vi "CopyOneBlock.vi"(8 "error in (no error)":errorcluster, 10 "block":u16) -> (0 "error out":errorcluster, 1 "data 2":u16[](array[numeric]), 2 "data 1":u16[](array[numeric]))   [LabVIEW 2015, in "ESLSCDLL.lvlib"]
uses:
  ESLSCDLL.lvlib
  Globals.vi
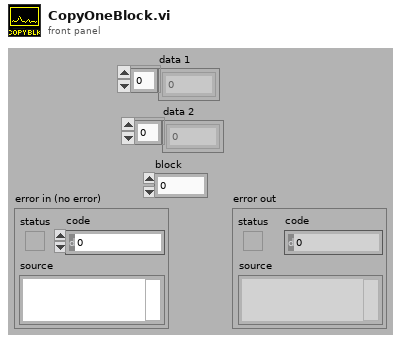
[diagram p1: front panel]
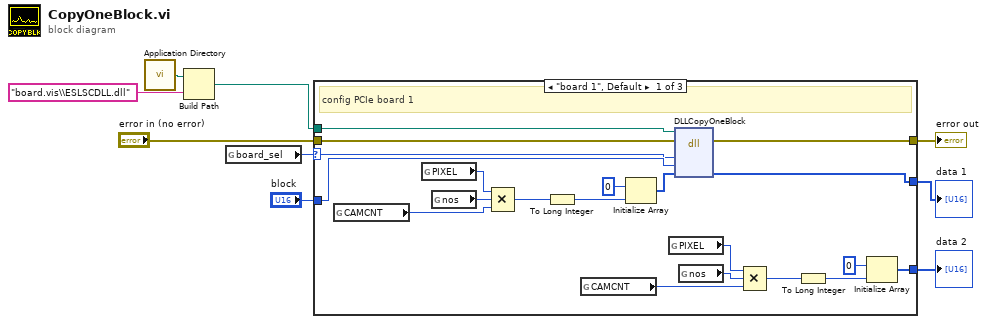
[diagram p0: block diagram]
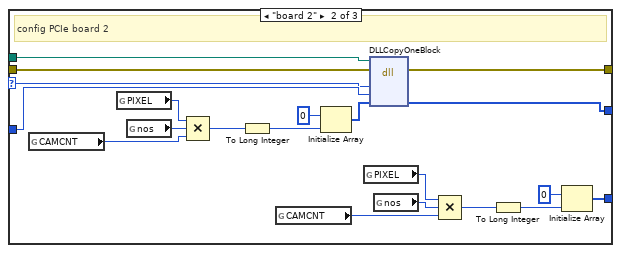
[diagram p2: hidden frame]
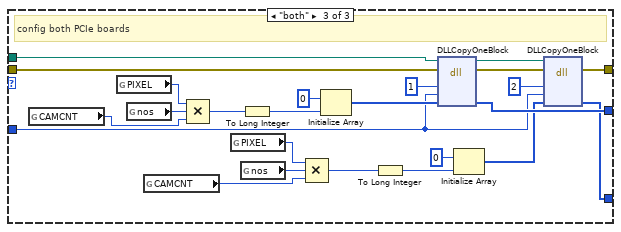
[diagram p3: hidden frame]
diagram:
  n1 = call <vilib>:"Application Directory.vi"() -> ("Application Directory"=w3:path)
  n2 = Build Path(base path=w3, name or relative path="board.vis\\ESLSCDLL.dll") -> (appended path=w1:path)
  n3 = global read "Globals.vi" "board_sel"() -> (w4:enum32{"0", "board 1", "board 2", "both"})
  n4 = case shown="\"board 1\", Default" w4 {
    selector: w4 -> [w20 w35 _]
    tunnel: [w22 w33 w60] -> w7
    tunnel: [w13 w34 w59] -> w9
    tunnel: "block" -> [w21 w36 w55]
    tunnel: "error in (no error)" -> [w12 w32 w54]
    tunnel: [w11 w31 w52] -> w5
    tunnel: w1 -> [w10 w30 w51]
    frame "board 1", Default {
      # "config PCIe board 1"
      n5 = global read "Globals.vi" "CAMCNT"() -> (w25:u32)
      n6 = global read "Globals.vi" "PIXEL"() -> (w26:u32)
      n7 = global read "Globals.vi" "nos"() -> (w24:u32)
      n8 = Compound Arithmetic op=MULTIPLY(w26, w24, w25) -> (w27:u32)
      n9 = To Long Integer(number=w27) -> (32bit integer=w29:i32)
      n10 = global read "Globals.vi" "CAMCNT"() -> (w15:u32)
      n11 = Initialize Array(u16 0, w29) -> (w23:u16[])
      n12 = global read "Globals.vi" "PIXEL"() -> (w16:u32)
      n13 = dll-call lib="C:/ENTW/PCIE/LV64/board.vis/ESLSCDLL.dll" fn="DLLCopyOneBlock" ("lwlscdll.dll:DLLReadLongS0")(path in=w10, error in=w12, "drv"=w20, "block"=w21, "pdest"=w23) -> (error out=w11:errorcluster, "pdest"=w22:u16[])  [unwired: 4 in, 1 out]
      n14 = global read "Globals.vi" "nos"() -> (w14:u32)
      n15 = Compound Arithmetic op=MULTIPLY(w16, w14, w15) -> (w17:u32)
      n16 = To Long Integer(number=w17) -> (32bit integer=w19:i32)
      n17 = Initialize Array(u16 0, w19) -> (w13:u16[])
    }
    frame "board 2" {
      # "config PCIe board 2"
      n18 = global read "Globals.vi" "CAMCNT"() -> (w45:u32)
      n19 = global read "Globals.vi" "PIXEL"() -> (w46:u32)
      n20 = global read "Globals.vi" "nos"() -> (w44:u32)
      n21 = Compound Arithmetic op=MULTIPLY(w46, w44, w45) -> (w47:u32)
      n22 = To Long Integer(number=w47) -> (32bit integer=w49:i32)
      n23 = global read "Globals.vi" "CAMCNT"() -> (w38:u32)
      n24 = Initialize Array(u16 0, w49) -> (w43:u16[])
      n25 = global read "Globals.vi" "PIXEL"() -> (w39:u32)
      n26 = dll-call lib="C:/ENTW/PCIE/LV64/board.vis/ESLSCDLL.dll" fn="DLLCopyOneBlock" ("lwlscdll.dll:DLLReadLongS0")(path in=w30, error in=w32, "drv"=w35, "block"=w36, "pdest"=w43) -> (error out=w31:errorcluster, "pdest"=w33:u16[])  [unwired: 4 in, 1 out]
      n27 = global read "Globals.vi" "nos"() -> (w37:u32)
      n28 = Compound Arithmetic op=MULTIPLY(w39, w37, w38) -> (w40:u32)
      n29 = To Long Integer(number=w40) -> (32bit integer=w42:i32)
      n30 = Initialize Array(u16 0, w42) -> (w34:u16[])
    }
    frame "both" {
      # "config both PCIe boards"
      n31 = global read "Globals.vi" "CAMCNT"() -> (w69:u32)
      n32 = global read "Globals.vi" "PIXEL"() -> (w70:u32)
      n33 = global read "Globals.vi" "nos"() -> (w68:u32)
      n34 = global read "Globals.vi" "CAMCNT"() -> (w62:u32)
      n35 = Compound Arithmetic op=MULTIPLY(w70, w68, w69) -> (w71:u32)
      n36 = global read "Globals.vi" "PIXEL"() -> (w63:u32)
      n37 = global read "Globals.vi" "nos"() -> (w61:u32)
      n38 = To Long Integer(number=w71) -> (32bit integer=w73:i32)
      n39 = Compound Arithmetic op=MULTIPLY(w63, w61, w62) -> (w64:u32)
      n40 = Initialize Array(u16 0, w73) -> (w67:u16[])
      n41 = To Long Integer(number=w64) -> (32bit integer=w66:i32)
      n42 = dll-call lib="C:/ENTW/PCIE/LV64/board.vis/ESLSCDLL.dll" fn="DLLCopyOneBlock" ("lwlscdll.dll:DLLReadLongS0")(path in=w51, error in=w54, "drv"=u32 1, "block"=w55, "pdest"=w67) -> (path out=w50:path, error out=w53:errorcluster, "pdest"=w60:u16[])  [unwired: 4 in]
      n43 = Initialize Array(u16 0, w66) -> (w58:u16[])
      n44 = dll-call lib="C:/ENTW/PCIE/LV64/board.vis/ESLSCDLL.dll" fn="DLLCopyOneBlock" ("lwlscdll.dll:DLLReadLongS0")(path in=w50, error in=w53, "drv"=u32 2, "block"=w55, "pdest"=w58) -> (error out=w52:errorcluster, "pdest"=w59:u16[])  [unwired: 4 in, 1 out]
    }
  }
  "data 1" <- w7
  "data 2" <- w9
  "error out" <- w5
